vi "Connector 0 AI.vi"() -> (3 "Packet":u64)   [LabVIEW 2014]
uses:
  <vilib>/rvi/eio/common/nirviEmuTemplateMethod_errors.vi
  <vilib>/eio/EIONode/EIONode.xnode
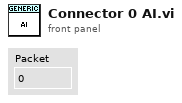
[diagram p1: front panel]
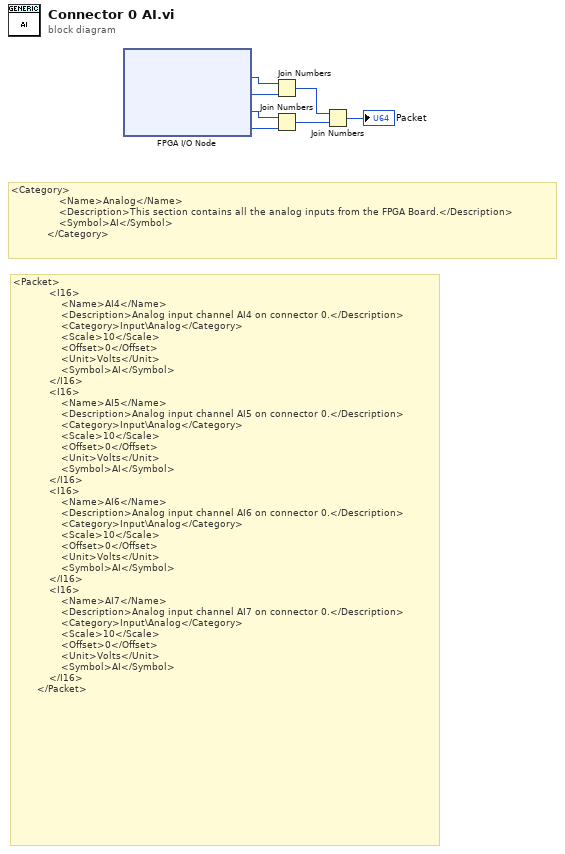
[diagram p0: block diagram]
diagram:
  # "<Packet>\n            <I16>\n                <Name>AI4</Name>\n                <Description>Analog input channel AI4 on connector 0.</Description>\n                <Category>Input\\Analog</Category>\n                <Scale>10</Scale>\n                <Offset>0</Offset>\n                <Unit>Volts</Unit>\n                <Symbol>AI</Symbol>\n            </I16>\n            <I16>\n                <Name>AI5</Name>\n                <Description>Analog input channel AI5 on connector 0.</Description>\n                <Category>Input\\Analog</Category>\n                <Scale>10</Scale>\n                <Offset>0</Offset>\n                <Unit>Volts</Unit>\n                <Symbol>AI</Symbol>\n            </I16>\n            <I16>\n                <Name>AI6</Name>\n                <Description>Analog input channel AI6 on connector 0.</Description>\n                <Category>Input\\Analog</Category>\n                <Scale>10</Scale>\n                <Offset>0</Offset>\n                <Unit>Volts</Unit>\n                <Symbol>AI</Symbol>\n            </I16>\n            <I16>\n                <Name>AI7</Name>\n                <Description>Analog input channel AI7 on connector 0.</Description>\n                <Category>Input\\Analog</Category>\n                <Scale>10</Scale>\n                <Offset>0</Offset>\n                <Unit>Volts</Unit>\n                <Symbol>AI</Symbol>\n            </I16>\n        </Packet>"
  # "<Category>\n                <Name>Analog</Name>\n                <Description>This section contains all the analog inputs from the FPGA Board.</Description>\n                <Symbol>AI</Symbol>\n            </Category>"
  n1 = xnode "FPGA I/O Node"() -> ("Connector0/AI7"=w3:i16, "Connector0/AI6"=w4:i16, "Connector0/AI5"=w5:i16, "Connector0/AI4"=w6:i16)  [unwired: 4 in, 4 out]
  n2 = Join Numbers(hi=w3, lo=w4) -> ((hi.lo)=w1:u32)
  n3 = Join Numbers(hi=w5, lo=w6) -> ((hi.lo)=w2:u32)
  n4 = Join Numbers(hi=w1, lo=w2) -> ((hi.lo)=→"Packet":u64)
